vi "trig -- arctan.vi"(0 "omega (kHz)":dbl, 1 "time in Gamma (sec)":dbl, 2 "delta t (sec)":dbl, 5 "gamma (kHz)":dbl, 12 "omega minus (kHz)":dbl, 13 "omega zero (kHz)":dbl, 14 "omega plus (kHz)":dbl) -> (4 "freq step (Hz)":dbl)   [LabVIEW 2015]
uses:
  Q - not nan -- real.vi
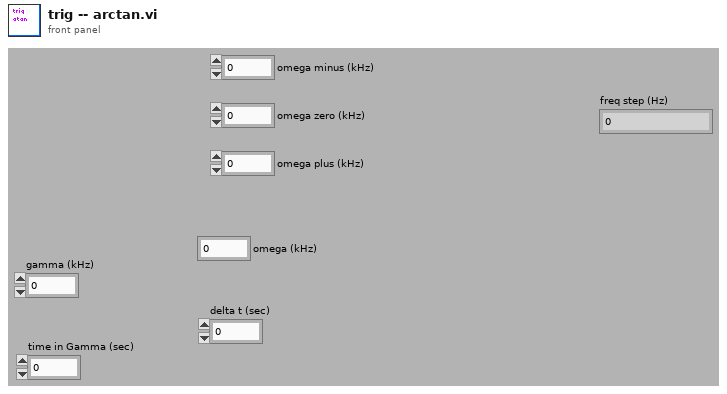
[diagram p1: front panel]
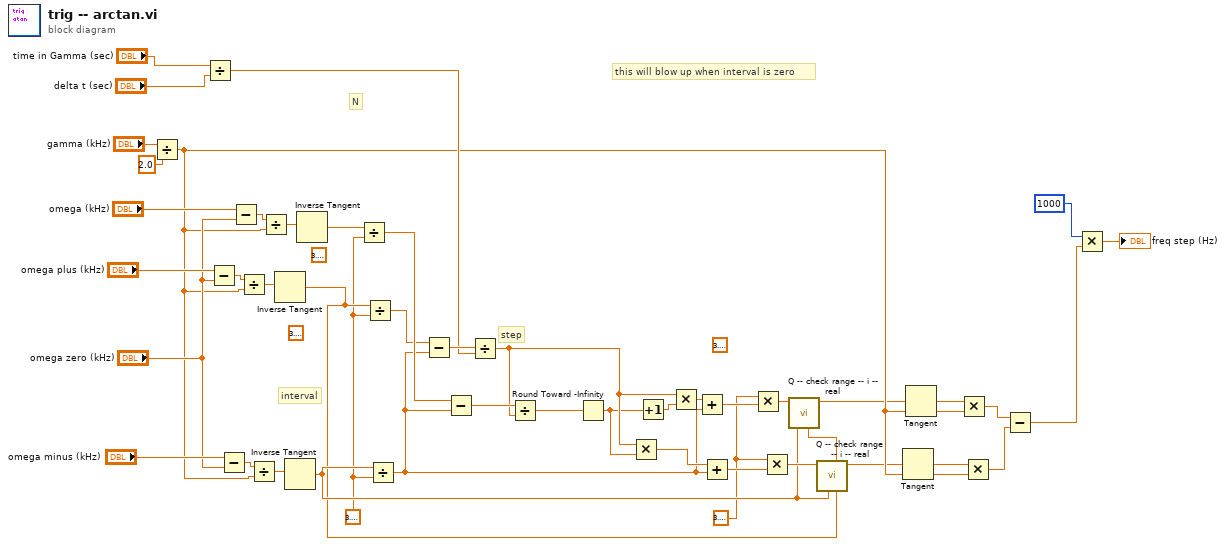
[diagram p0: block diagram]
diagram:
  w1 = 3.141592653589793
  (unwired) 3.141592653589793
  w2 = 3.141592653589793
  (unwired) 3.141592653589793
  (unwired) 3.141592653589793
  # "this will blow up when interval is zero"
  # "interval"
  # "step"
  # "N"
  n1 = Divide(x="gamma (kHz)", y=2.0) -> (x/y=w22:dbl)
  n2 = Divide(x="time in Gamma (sec)", y="delta t (sec)") -> (x/y=w34:dbl)
  n3 = Subtract(x="omega plus (kHz)", y="omega zero (kHz)") -> (x-y=w41:dbl)
  n4 = Subtract(x="omega minus (kHz)", y="omega zero (kHz)") -> (x-y=w43:dbl)
  n5 = Subtract(x="omega (kHz)", y="omega zero (kHz)") -> (x-y=w45:dbl)
  n6 = Divide(x=w41, y=w22) -> (x/y=w40:dbl)
  n7 = Divide(x=w43, y=w22) -> (x/y=w42:dbl)
  n8 = Divide(x=w45, y=w22) -> (x/y=w44:dbl)
  n9 = Inverse Tangent(1:w40) -> (0:w3:dbl)
  n10 = Inverse Tangent(1:w42) -> (0:w4:dbl)
  n11 = Inverse Tangent(1:w44) -> (0:w14:dbl)
  n12 = Divide(x=w14, y=w2) -> (x/y=w13:dbl)
  n13 = Divide(x=w3, y=w2) -> (x/y=w7:dbl)
  n14 = Divide(x=w4, y=w2) -> (x/y=w8:dbl)
  n15 = Subtract(x=w7, y=w8) -> (x-y=w35:dbl)
  n16 = Subtract(x=w13, y=w8) -> (x-y=w27:dbl)
  n17 = Divide(x=w35, y=w34) -> (x/y=w24:dbl)
  n18 = Divide(x=w27, y=w24) -> (x/y=w26:dbl)
  n19 = Round Toward -Infinity(1:w26) -> (0:w18:dbl)
  n20 = Multiply(x=w24, y=w18) -> (x*y=w17:dbl)
  n21 = Increment(x=w18) -> (x+1=w16:dbl)
  n22 = Multiply(x=w24, y=w16) -> (x*y=w15:dbl)
  n23 = Add(x=w15, y=w8) -> (x+y=w12:dbl)
  n24 = Add(x=w17, y=w8) -> (x+y=w11:dbl)
  n25 = Multiply(x=w1, y=w12) -> (x*y=w10:dbl)
  n26 = Multiply(x=w1, y=w11) -> (x*y=w6:dbl)
  n27 = call "Q -- check range -- i -- real.vi"("upper"=w3, "lower"=w4, "number"=w10) -> ("number in range"=w9:dbl)  [unwired: 6 in, 2 out]
  n28 = call "Q -- check range -- i -- real.vi"("upper"=w3, "lower"=w4, "number"=w6) -> ("number in range"=w5:dbl)  [unwired: 6 in, 2 out]
  n29 = Tangent(1:w5) -> (0:w23:dbl)
  n30 = Tangent(1:w9) -> (0:w25:dbl)
  n31 = Multiply(x=w25, y=w22) -> (x*y=w21:dbl)
  n32 = Multiply(x=w23, y=w22) -> (x*y=w20:dbl)
  n33 = Subtract(x=w21, y=w20) -> (x-y=w19:dbl)
  n34 = Multiply(x=1000 ("dimension size"), y=w19) -> (x*y=→"freq step (Hz)":dbl)
